vi "set AC test parameters.vi"(7 "AC Parameters":T1={"Voltage Level [V] "=1500, "Hi Limit [A]"=0.005, "Test Time [s] "=8.0, "Lo Limit [A]"=0.0001, "ARC Limit [A]"=0.005, "Ramp Time [s] "=1.1, "Fall Time [s]"=2.2} {"Voltage Level [V]" min=50 max=5000 step=1 format="%.3p"; "Hi Limit [A]" min=0.0001 max=0.03 step=1e-07 format="%.3p"; "Test Time [s]" min=0.0 max=999.0 step=0.1 format="%.1p"; "Lo Limit [A]" min=0.0 max=0.03 step=1e-07 format="%.3p"; "ARC Limit [A]" min=0.0 max=15.0 format="%.1p"; "Ramp Time [s]" min=0.0 max=999.0 step=0.1 format="%.1p"; "Fall Time [s]" min=0.0 max=999.0 step=0.1 format="%.1p"}, 8 "error in (no error)":errorcluster, 10 "Step":T2 min=1 max=99 step=1, 11 "VISA Refnum in":refnum<visa-resource-name>) -> (0 "error out":errorcluster, 3 "VISA Refnum out":refnum<visa-resource-name>)   [LabVIEW 2025]
uses:
  controls/Step--numeric.ctl
  setters & getters/AC parameters--cluster.ctl
  <instrlib>/Chrome 19025/Public/Utility/Type Def/AC-DC modes--ring.ctl
  <instrlib>/Chrome 19025/Public/Utility/Type Def/AC-DC-IR modes--ring.ctl
  <instrlib>/Chrome 19025/Chrome 19025.lvlib
panel:
  # "AC"
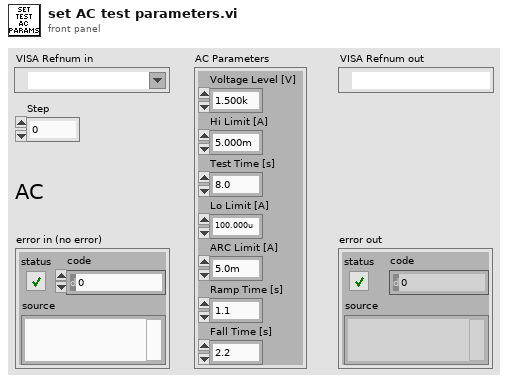
[diagram p1: front panel]
types:
  T1 = typedef "AC parameters--cluster.ctl" = cluster{"Voltage Level [V] ":u16, "Hi Limit [A]":dbl, "Test Time [s] ":dbl, "Lo Limit [A]":dbl, "ARC Limit [A]":dbl, "Ramp Time [s] ":dbl, "Fall Time [s]":dbl}
  T2 = typedef "Step--numeric.ctl" = u8
  T3 = typedef "Chrome 19025.lvlib/AC-DC modes--ring.ctl" = i32
  T4 = typedef "Chrome 19025.lvlib/AC-DC-IR modes--ring.ctl" = u16
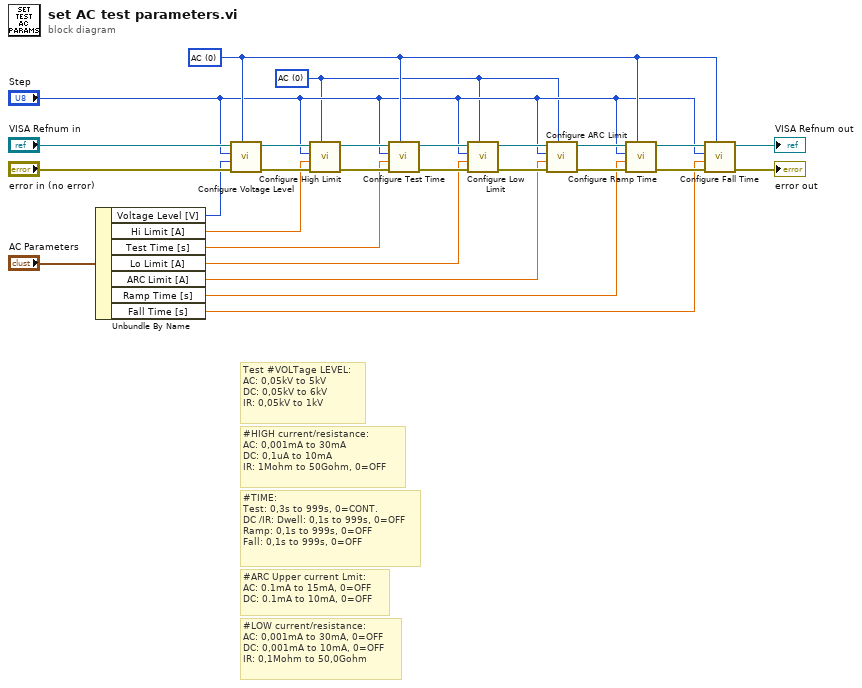
[diagram p0: block diagram]
diagram:
  w9 = T3 0 items=["AC", "DC"] ("Mode")
  w13 = T4 0 items=["AC", "DC", "IR"] ("Mode")
  # "#ARC Upper current Lmit:\nAC: 0.1mA to 15mA, 0=OFF\nDC: 0.1mA to 10mA, 0=OFF"
  # "#TIME: \nTest: 0,3s to 999s, 0=CONT. \nDC /IR: Dwell: 0,1s to 999s, 0=OFF\nRamp: 0,1s to 999s, 0=OFF\nFall: 0,1s to 999s, 0=OFF"
  # "#LOW current/resistance: \nAC: 0,001mA to 30mA, 0=OFF\nDC: 0,001mA to 10mA, 0=OFF\nIR: 0,1Mohm to 50,0Gohm"
  # "#HIGH current/resistance: \nAC: 0,001mA to 30mA\nDC: 0,1uA to 10mA\nIR: 1Mohm to 50Gohm, 0=OFF"
  # "Test #VOLTage LEVEL: \nAC: 0,05kV to 5kV\nDC: 0,05kV to 6kV\nIR: 0,05kV to 1kV"
  n1 = Unbundle By Name("AC Parameters") -> ("Voltage Level [V]"=w7:u16, "Hi Limit [A]"=w6:dbl, "Test Time [s]"=w5:dbl, "Lo Limit [A]"=w4:dbl, "ARC Limit [A]"=w3:dbl, "Ramp Time [s]"=w2:dbl, "Fall Time [s]"=w1:dbl)
  n2 = call <instrlib>:"Configure Voltage Level.vi"("Mode"=w13, "error in (no error)"="error in (no error)", "Voltage Level [V]"=w7, "Step"="Step", "VISA resource name"="VISA Refnum in") -> ("error out"=w19:errorcluster, "VISA resource name out"=w16:refnum<visa-resource-name>)  [unwired: 5 in]
  n3 = call <instrlib>:"Configure High Limit.vi"("Mode"=w9, "error in (no error)"=w19, "Hi Limit [A]"=w6, "Step"="Step", "VISA resource name"=w16) -> ("error out"=w26:errorcluster, "VISA resource name out"=w27:refnum<visa-resource-name>)  [unwired: 5 in]
  n4 = call <instrlib>:"Configure Test Time.vi"("Mode"=w13, "error in (no error)"=w26, "Test Time [s]"=w5, "Step"="Step", "VISA resource name"=w27) -> ("error out"=w15:errorcluster, "VISA resource name out"=w14:refnum<visa-resource-name>)  [unwired: 5 in]
  n5 = call <instrlib>:"Configure Low Limit.vi"("Mode"=w9, "error in (no error)"=w15, "Lo Limit [A]"=w4, "Step"="Step", "VISA resource name"=w14) -> ("error out"=w20:errorcluster, "VISA resource name out"=w21:refnum<visa-resource-name>)  [unwired: 5 in]
  n6 = call <instrlib>:"Configure ARC Limit.vi"("Mode"=w9, "error in (no error)"=w20, "ARC Limit [A]"=w3, "Step"="Step", "VISA resource name"=w21) -> ("error out"=w22:errorcluster, "VISA resource name out"=w24:refnum<visa-resource-name>)  [unwired: 5 in]
  n7 = call <instrlib>:"Configure Ramp Time.vi"("Mode"=w13, "error in (no error)"=w22, "Ramp Time [s]"=w2, "Step"="Step", "VISA resource name"=w24) -> ("error out"=w23:errorcluster, "VISA resource name out"=w25:refnum<visa-resource-name>)  [unwired: 5 in]
  n8 = call <instrlib>:"Configure Fall Time.vi"("Mode"=w13, "error in (no error)"=w23, "Fall Time [s]"=w1, "Step"="Step", "VISA resource name"=w25) -> ("error out"=→"error out":errorcluster, "VISA resource name out"=→"VISA Refnum out":refnum<visa-resource-name>)  [unwired: 5 in]
